vi "destroy.vi"(8 "error in (no error)":errorcluster, 11 "comic_crawler in":refnum<class "comic_crawler.lvclass">) -> (0 "error out":errorcluster)   [LabVIEW 2024, in "comic_crawler.lvclass"]
uses:
  comic_crawler.lvclass
  private/daemon.states--enum.ctl
  comic_crawler.lvclass/comic_crawler.ctl
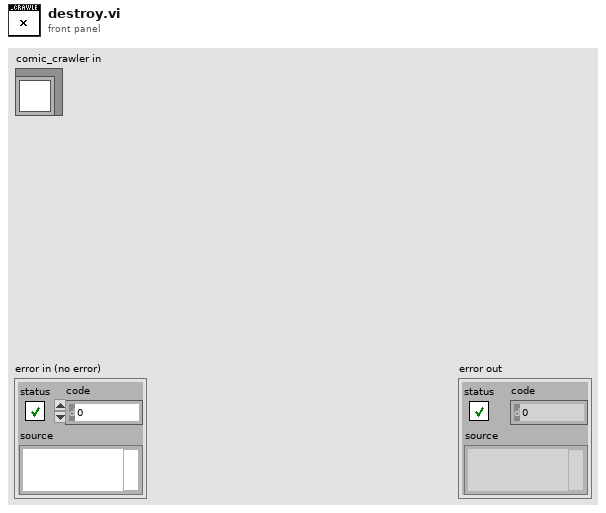
[diagram p1: front panel]
types:
  T1 = typedef "comic_crawler.lvclass/daemon.states--enum.ctl" = enum16{"start search", "idle", "set timer", "running", "stop search", "wait", "set delay", "shut down"}
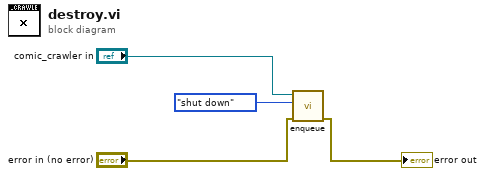
[diagram p0: block diagram]
diagram:
  n1 = call "enqueue.vi"("error in (no error)"="error in (no error)", "cmd"=daemon.states--enum."shut down", "comic_crawler in"="comic_crawler in") -> ("error out"=→"error out":errorcluster)  [unwired: 7 in, 1 out]
